vi "addSignal.vi"(8 "error in (no error)":errorcluster, 10 "ISignal in":refnum<class "ISignal.lvclass">, 11 "IMultiReaderBuilder in":refnum<class "IMultiReaderBuilder.lvclass">) -> (0 "error out":errorcluster, 2 "ISignal out":refnum<class "ISignal.lvclass">, 3 "IMultiReaderBuilder out":refnum<class "IMultiReaderBuilder.lvclass">, 4 "return type":u32)   [LabVIEW 2022 SP3, in "openDAQ.lvlib" / "IBaseObject.lvlib" / "IMultiReaderBuilder.lvlib" / "IMultiReaderBuilder.lvclass"]
uses:
  <instrlib>/openDAQ/Public/Classes/IMultiReaderBuilder/IMultiReaderBuilder.lvclass
  C:/Program Files (x86)/National Instruments/LabVIEW 2022/instr.lib/openDAQ/Public/Classes/IBaseObject/IBaseObject.lvclass
  <instrlib>/openDAQ/Public/Classes/ISignal/ISignal.lvclass
  <instrlib>/openDAQ/Public/Classes/IBaseObject/IBaseObject.lvclass/IBaseObject.ctl
  <instrlib>/openDAQ/Public/Classes/IBaseObject/Accessor/Read reference.vi
  <instrlib>/openDAQ/Public/Classes/IBaseObject/Accessor/Write reference.vi
  <instrlib>/openDAQ/Binaries/Windows/x86/copendaq32.dll
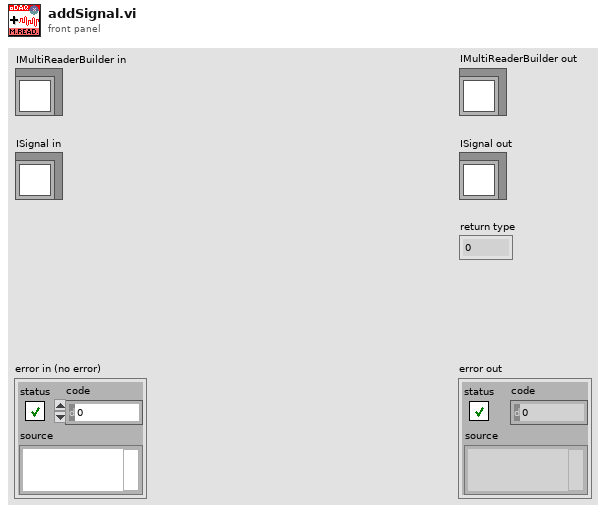
[diagram p1: front panel]
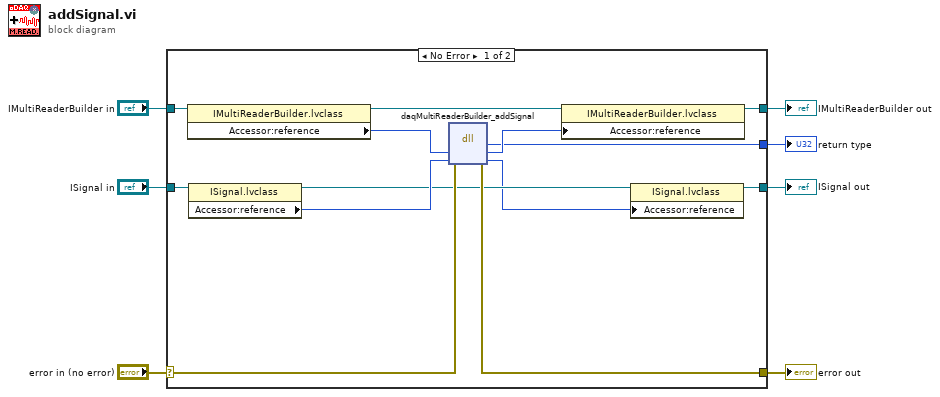
[diagram p0: block diagram]
diagram:
  n1 = case shown="No Error" "error in (no error)" {
    selector: "error in (no error)" -> [w18 w23]
    tunnel: [w17 w23] -> w6
    tunnel: [w15 w22] -> w4
    tunnel: "IMultiReaderBuilder in" -> [w19 w22]
    tunnel: "ISignal in" -> [w12 w21]
    tunnel: [w10 w21] -> w2
    tunnel: [w8 _] -> w1
    frame No Error {
      n2 = property class="IMultiReaderBuilder.lvclass"(reference=w19) -> (reference out=w16:refnum<class "IMultiReaderBuilder.lvclass">, "Accessor:reference"=w14:i64)  [unwired: 1 in, 1 out]
      n3 = property class="ISignal.lvclass"(reference=w12) -> (reference out=w11:refnum<class "ISignal.lvclass">, "Accessor:reference"=w20:i64)  [unwired: 1 in, 1 out]
      n4 = dll-call lib="C:/Program Files (x86)/National Instruments/LabVIEW 2022/instr.lib/openDAQ/Binaries/Windows/x86/copendaq*.*" fn="daqMultiReaderBuilder_addSignal"(error in=w18, "builder"=w14, "signal"=w20) -> (error out=w17:errorcluster, "return type"=w8:u32, "builder"=w13:i64, "signal"=w9:i64)  [unwired: 2 in, 1 out]
      n5 = property class="IMultiReaderBuilder.lvclass"(reference=w16, "Accessor:reference"=w13) -> (reference out=w15:refnum<class "IMultiReaderBuilder.lvclass">)  [unwired: 1 in, 1 out]
      n6 = property class="ISignal.lvclass"(reference=w11, "Accessor:reference"=w9) -> (reference out=w10:refnum<class "ISignal.lvclass">)  [unwired: 1 in, 1 out]
    }
    frame Error {
    }
  }
  "error out" <- w6
  "IMultiReaderBuilder out" <- w4
  "ISignal out" <- w2
  "return type" <- w1
